vi "Convert_Graph_HD_v00.vi"(8 "Extras Homodyne":T1, 11 "PII Control":T2={"Pre-Offset p Error"=-0.08983050847457627, "Gain Error x"=1, "P Gain"=0, "P Bit Shift"=1, "I Bit Shift"=20, "I2 Bit Shift"=-12, "I Gain"=-12, "I2 Gain"=-27, "Lock Threshold"=20, "Lock"=FALSE, "Hold"=FALSE, "Scan Frequency"=8, "Scan Bit Shift"=-5, "Gains -ve "=TRUE, "Pre- Offset x"=-4.0, "Lock Angle (ƒÆ)"=0.0, "Gain Error p\n\n"=1} {"Lock Angle (ƒÆ)" min=-90.0 max=90.0 scale=-90.0..90.0 scale format="%#_2g"; "Pre- Offset x" scale=-0.01..0.01 scale format="%#_5f"; "Scan Frequency" scale=1.0..30.0; "I2 Gain" scale=0.0..10.0; "I Gain" scale=0.0..50.0; "P Gain" scale=0.0..50.0; "Pre-Offset p Error" scale=-0.01..0.01 scale format="%#_5f"}) -> (3 "PII+Error":T12)   [LabVIEW 2010]
uses:
  Strict Type Defs/PII individual.ctl
  Strict Type Defs/Errors Converted Graph HD.ctl
  Strict Type Defs/PII and Error Graph HD.ctl
  Strict Type Defs/GUI HD Graph.ctl
  Strict Type Defs/Slider and display.ctl
  Strict Type Defs/I16 white control.ctl
  Strict Type Defs/PII Gains.ctl
  Strict Type Defs/I2 gain slider.ctl
  Strict Type Defs/Thresh slider.ctl
  Strict Type Defs/Lock or Hold.ctl
  Strict Type Defs/Scan Freq Slider.ctl
  Strict Type Defs/Gains negative vertical.ctl
  Strict Type Defs/theta.ctl
  Strict Type Defs/Extras PII Graph HD.ctl
panel:
  in  "PII+Error type def":T12
  in  "Error individual":T13
  in  "PII In typdef":T14
  # "PII Gains"
  # "Lock"
  # "Error Signal"
  # "Scan"
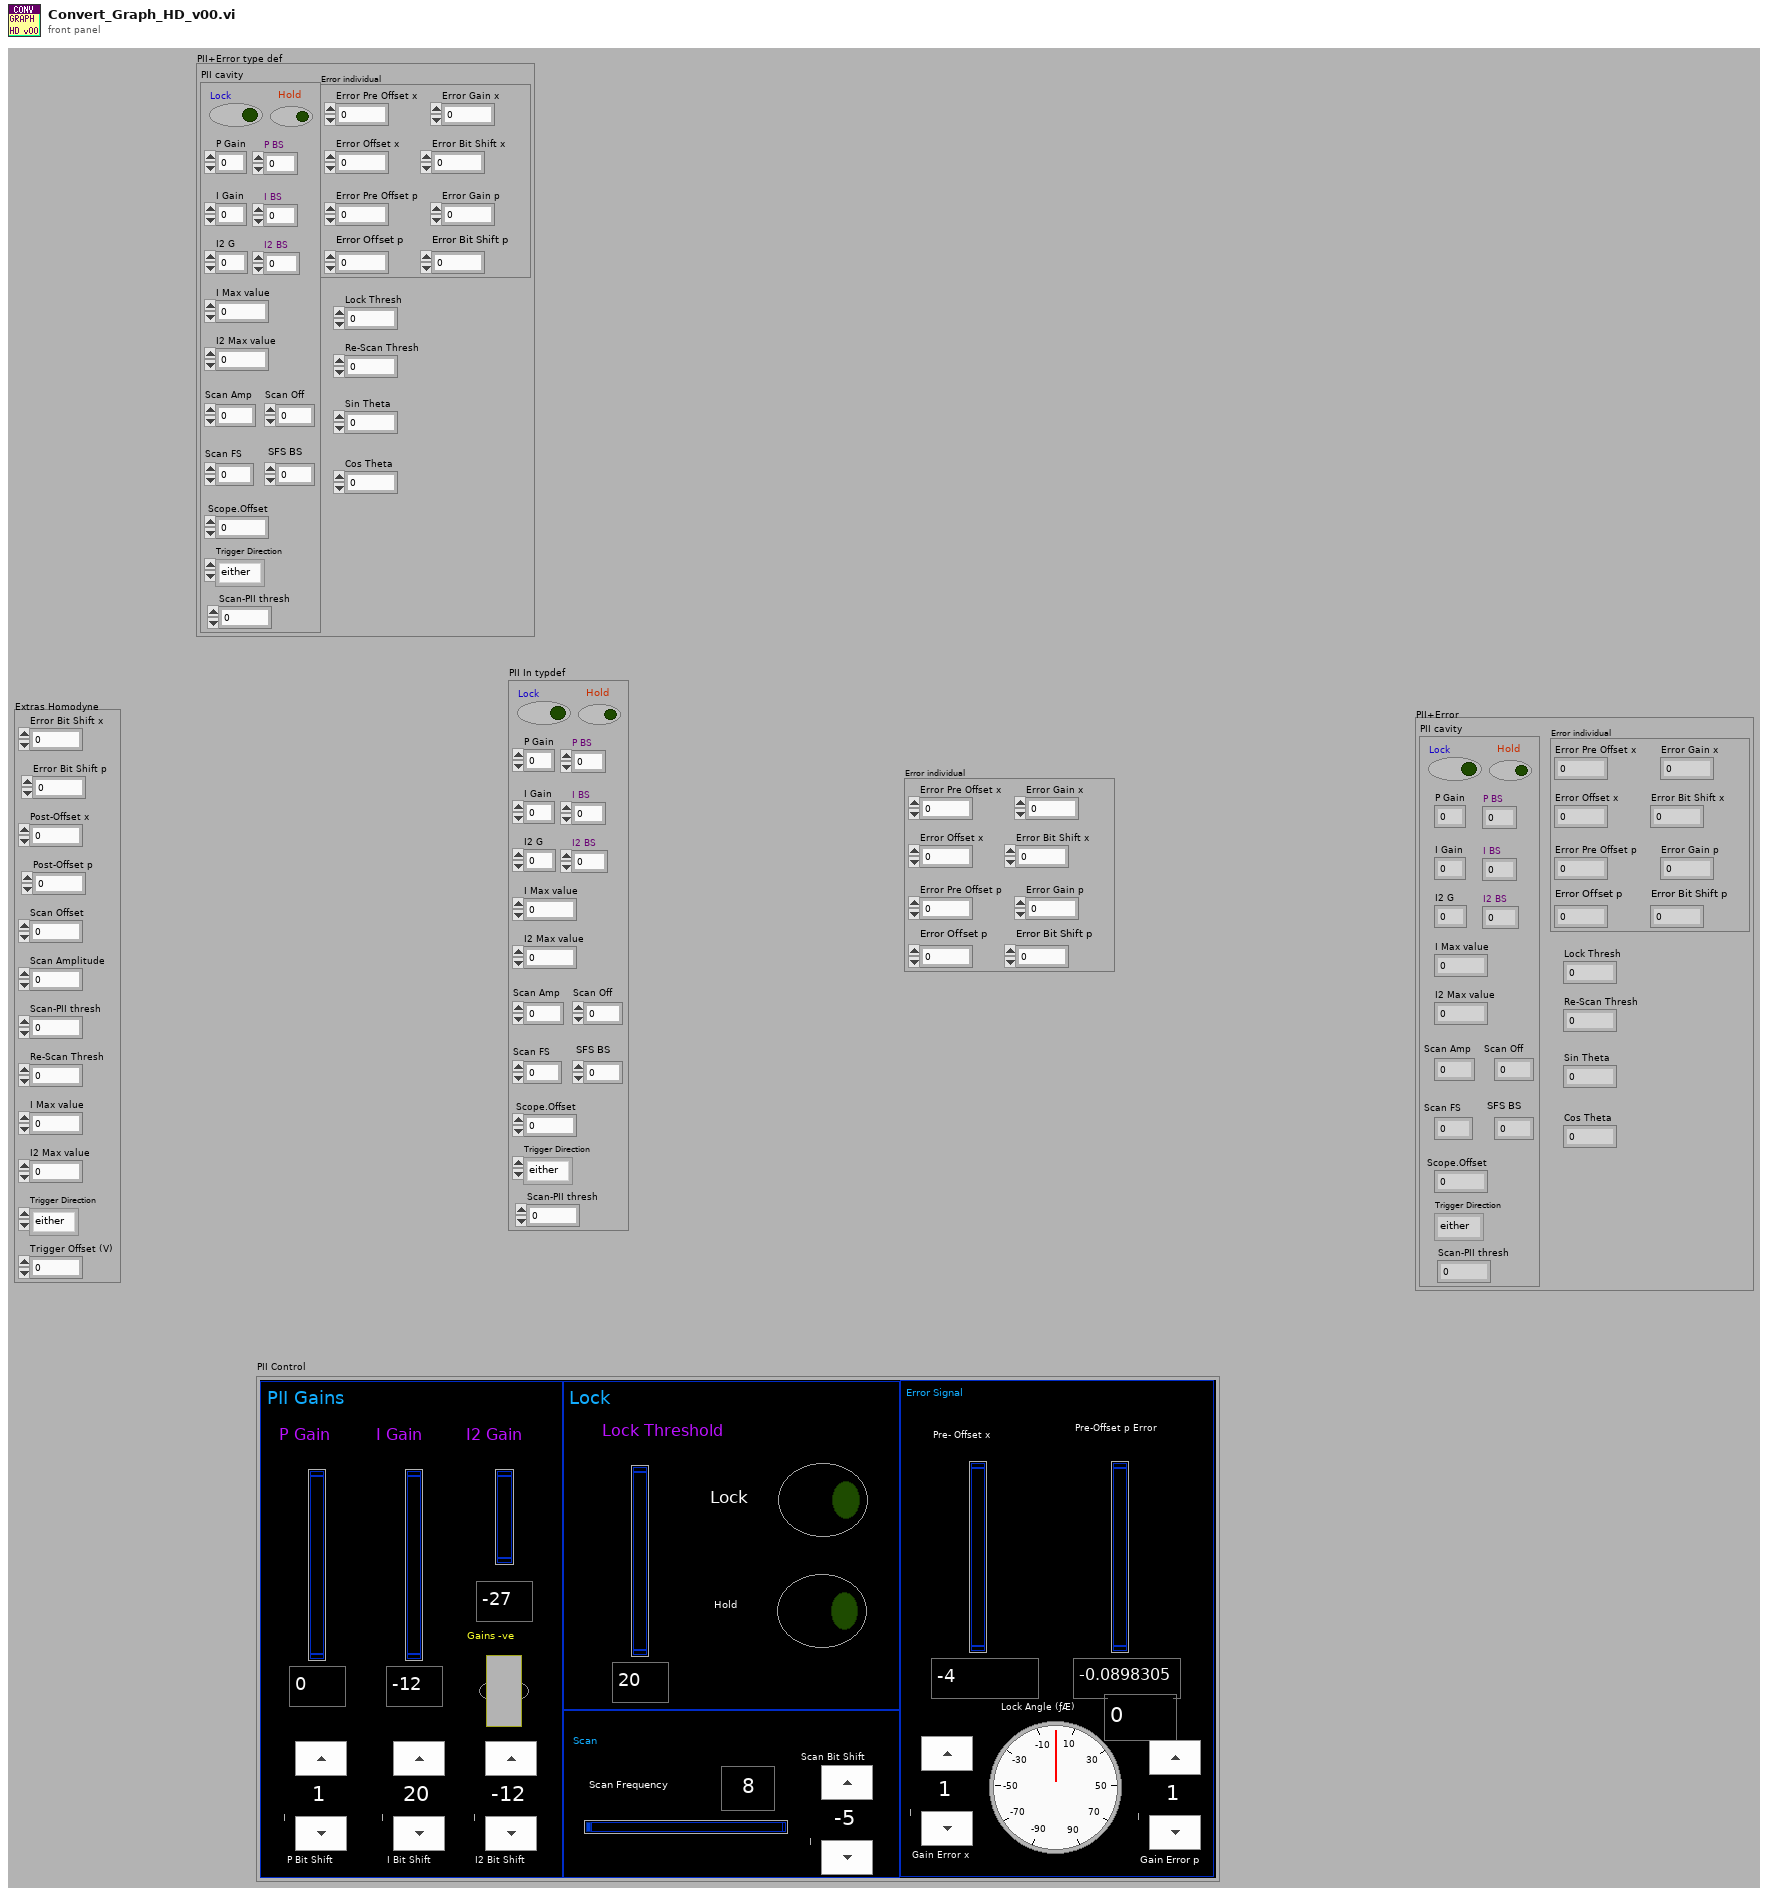
[diagram p1: front panel]
types:
  T1 = typedef "Extras PII Graph HD.ctl" = cluster{"Error Bit Shift p":i16, "Scan Offset":dbl, "Scan Amplitude":dbl, "Scan-PII thresh":i16, "Re-Scan Thresh":i16, "I Max value":i32, "I2 Max value":i32, "Trigger Direction":enum8{"either", "minus-plus", "plus-minus"}, "Trigger Offset (V)":dbl, "Error Bit Shift x":i16, "Post-Offset p":dbl, "Post-Offset x":dbl}
  T2 = typedef "GUI HD Graph.ctl" = cluster{"Pre-Offset p Error":T3, "Gain Error x":T4, "P Gain":T5, "P Bit Shift":T4, "I Bit Shift":T4, "I2 Bit Shift":T4, "I Gain":T5, "I2 Gain":T6, "Lock Threshold":T7, "Lock":T8, "Hold":T8, "Scan Frequency":T9, "Scan Bit Shift":T4, "Gains -ve ":T10, "Pre- Offset x":T3, "Lock Angle (ƒÆ)":T11, "Gain Error p\n\n":T4}
  T3 = typedef "Slider and display.ctl" = dbl
  T4 = typedef "I16 white control.ctl" = i16
  T5 = typedef "PII Gains.ctl" = i32
  T6 = typedef "I2 gain slider.ctl" = i32
  T7 = typedef "Thresh slider.ctl" = i16
  T8 = typedef "Lock or Hold.ctl" = bool
  T9 = typedef "Scan Freq Slider.ctl" = u16
  T10 = typedef "Gains negative vertical.ctl" = bool
  T11 = typedef "theta.ctl" = dbl
  T12 = typedef "PII and Error Graph HD.ctl" = cluster{"Error individual":T13, "PII cavity":T14, "Lock Thresh":i16, "Re-Scan Thresh":i16, "Sin Theta":i32, "Cos Theta":i32}
  T13 = typedef "Errors Converted Graph HD.ctl" = cluster{"Error Pre Offset x":i16, "Error Offset x":i16, "Error Gain x":i16, "Error Bit Shift x":i16, "Error Pre Offset p":i16, "Error Offset p":i16, "Error Gain p":i16, "Error Bit Shift p":i16}
  T14 = typedef "PII individual.ctl" = cluster{"Lock":bool, "Hold":bool, "P Gain":i32, "P BS":i16, "I Gain":i32, "I BS":i16, "I2 G":i32, "I2 BS":i16, "Scan Amp":i16, "Scan Off":i16, "Scan FS":u16, "SFS BS":i16, "I Max value":i32, "I2 Max value":i32, "Scope.Offset":i16, "Trigger Direction":enum8{"either", "minus-plus", "plus-minus"}, "Scan-PII thresh":i16}
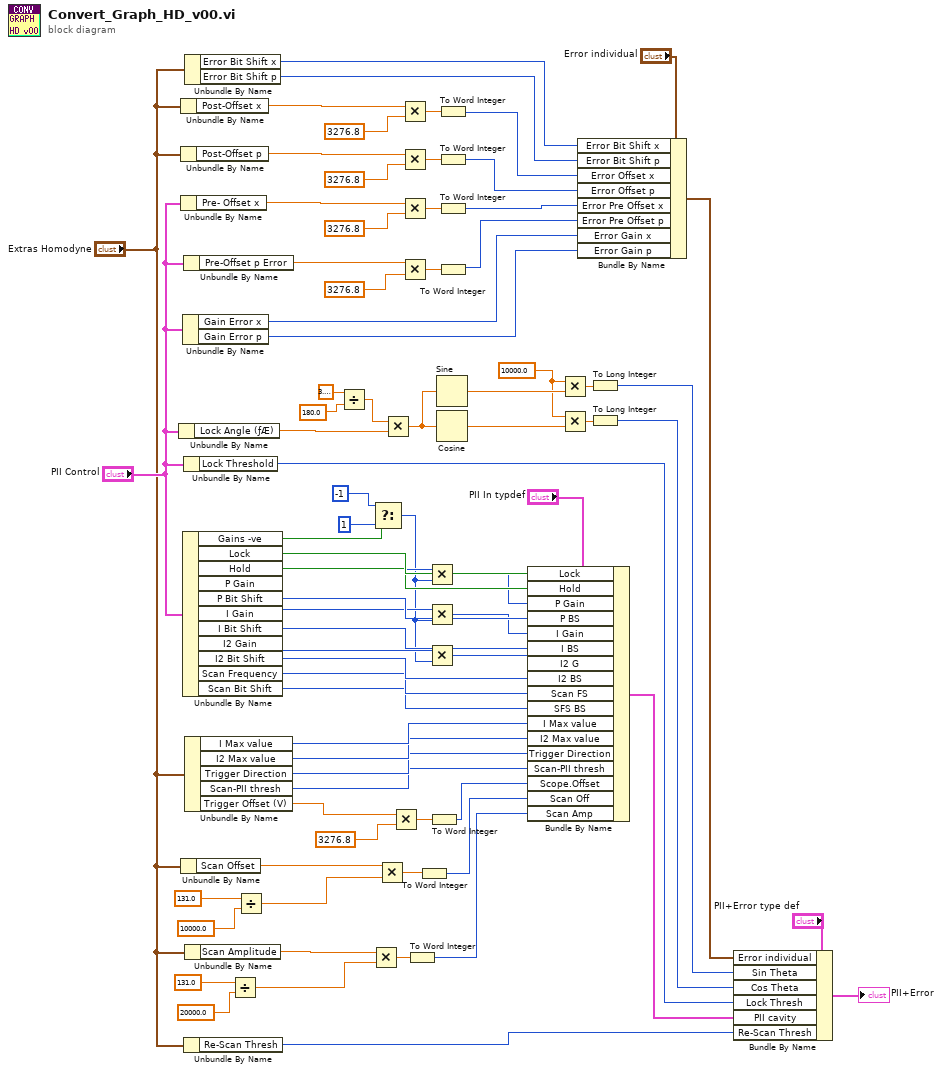
[diagram p0: block diagram]
diagram:
  w17 = T11 10000.0 ("x")
  n1 = Unbundle By Name("PII Control") -> ("Lock Angle (ƒÆ)"=w21:T11)
  n2 = Unbundle By Name("Extras Homodyne") -> ("Post-Offset x"=w8:dbl)
  n3 = Unbundle By Name("Extras Homodyne") -> ("Post-Offset p"=w6:dbl)
  n4 = Unbundle By Name("PII Control") -> ("Pre- Offset x"=w13:T3)
  n5 = Unbundle By Name("Extras Homodyne") -> ("Scan Offset"=w40:dbl)
  n6 = Unbundle By Name("PII Control") -> ("Gain Error x"=w42:T4, "Gain Error p"=w1:T4)
  n7 = Unbundle By Name("PII Control") -> ("Gains -ve"=w59:T10, "Lock"=w64:T8, "Hold"=w63:T8, "P Gain"=w58:T5, "P Bit Shift"=w62:T4, "I Gain"=w54:T5, "I Bit Shift"=w61:T4, "I2 Gain"=w52:T6, "I2 Bit Shift"=w60:T4, "Scan Frequency"=w49:T9, "Scan Bit Shift"=w48:T4)
  n8 = Unbundle By Name("PII Control") -> ("Pre-Offset p Error"=w75:T3)
  n9 = Unbundle By Name("PII Control") -> ("Lock Threshold"=w39:T7)
  n10 = Unbundle By Name("Extras Homodyne") -> ("Re-Scan Thresh"=w28:i16)
  n11 = Unbundle By Name("Extras Homodyne") -> ("Error Bit Shift x"=w11:i16, "Error Bit Shift p"=w12:i16)
  n12 = Unbundle By Name("Extras Homodyne") -> ("I Max value"=w37:i32, "I2 Max value"=w36:i32, "Trigger Direction"=w35:enum8{"either", "minus-plus", "plus-minus"}, "Scan-PII thresh"=w34:i16, "Trigger Offset (V)"=w30:dbl)
  n13 = Unbundle By Name("Extras Homodyne") -> ("Scan Amplitude"=w74:dbl)
  n14 = Divide(x=131.0, y=20000.0) -> (x/y=w69:dbl)
  n15 = Divide(x=131.0, y=10000.0) -> (x/y=w66:dbl)
  n16 = Divide(x=3.141592653589793, y=180.0) -> (x/y=w22:dbl)
  n17 = Multiply(x=w74, y=w69) -> (x*y=w72:dbl)
  n18 = Select(t=T5 -1 ("y"), s=w59, f=T5 1) -> (s? t:f=w50:T5)
  n19 = Multiply(x=w40, y=w66) -> (x*y=w73:dbl)
  n20 = Multiply(x=w22, y=w21) -> (x*y=w25:T11)
  n21 = Multiply(x=w30, y=3276.8) -> (x*y=w32:dbl)
  n22 = Multiply(x=w8, y=3276.8) -> (x*y=w10:dbl)
  n23 = Multiply(x=w6, y=3276.8) -> (x*y=w4:dbl)
  n24 = Multiply(x=w13, y=3276.8) -> (x*y=w78:T3)
  n25 = Multiply(x=w75, y=3276.8) -> (x*y=w77:T3)
  n26 = To Word Integer(number=w72) -> (16bit integer=w38:i16)
  n27 = To Word Integer(number=w73) -> (16bit integer=w33:i16)
  n28 = Multiply(x=w58, y=w50) -> (x*y=w55:T5)
  n29 = Multiply(x=w54, y=w50) -> (x*y=w53:T5)
  n30 = Multiply(x=w52, y=w50) -> (x*y=w51:T6)
  n31 = To Word Integer(number=w32) -> (16bit integer=w29:i16)
  n32 = Sine(x=w25) -> (sin(x)=w20:T11)
  n33 = Cosine(x=w25) -> (cos(x)=w18:T11)
  n34 = To Word Integer(number=w10) -> (16bit integer=w7:i16)
  n35 = To Word Integer(number=w4) -> (16bit integer=w2:i16)
  n36 = To Word Integer(number=w78) -> (16bit integer=w46:i16)
  n37 = To Word Integer(number=w77) -> (16bit integer=w45:i16)
  n38 = Bundle By Name(cluster="PII In typdef", "Lock"=w64, "Hold"=w63, "P Gain"=w55, "P BS"=w62, "I Gain"=w53, "I BS"=w61, "I2 G"=w51, "I2 BS"=w60, "Scan FS"=w49, "SFS BS"=w48, "I Max value"=w37, "I2 Max value"=w36, "Trigger Direction"=w35, "Scan-PII thresh"=w34, "Scope.Offset"=w29, "Scan Off"=w33, "Scan Amp"=w38) -> (w43:T14)
  n39 = Multiply(x=w17, y=w20) -> (x*y=w26:T11)
  n40 = Multiply(x=w17, y=w18) -> (x*y=w19:T11)
  n41 = Bundle By Name(cluster="Error individual", "Error Bit Shift x"=w11, "Error Bit Shift p"=w12, "Error Offset x"=w7, "Error Offset p"=w2, "Error Pre Offset x"=w46, "Error Pre Offset p"=w45, "Error Gain x"=w42, "Error Gain p"=w1) -> (w27:T13)
  n42 = To Long Integer(number=w26) -> (32bit integer=w15:i32)
  n43 = To Long Integer(number=w19) -> (32bit integer=w16:i32)
  n44 = Bundle By Name(cluster="PII+Error type def", "Error individual"=w27, "Sin Theta"=w15, "Cos Theta"=w16, "Lock Thresh"=w39, "PII cavity"=w43, "Re-Scan Thresh"=w28) -> (→"PII+Error":T12)
